vi "Execute FlatSeqOutTun Handle.vi"(6 "Menu Item Tag Suffix":string, 8 "错误输入（无错误）":errorcluster, 11 "平铺式顺序外部隧道输入":refnum<vi>) -> (0 "错误输出":errorcluster)   [LabVIEW 2020]
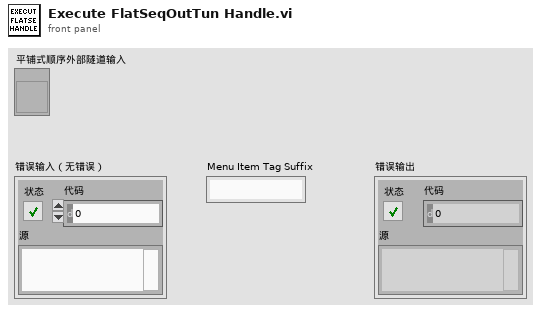
[diagram p1: front panel]
types:
  T1 = typedef "LVRectTypeDef.ctl" = cluster{"Left":i16, "Top":i16, "Right":i16, "Bottom":i16}
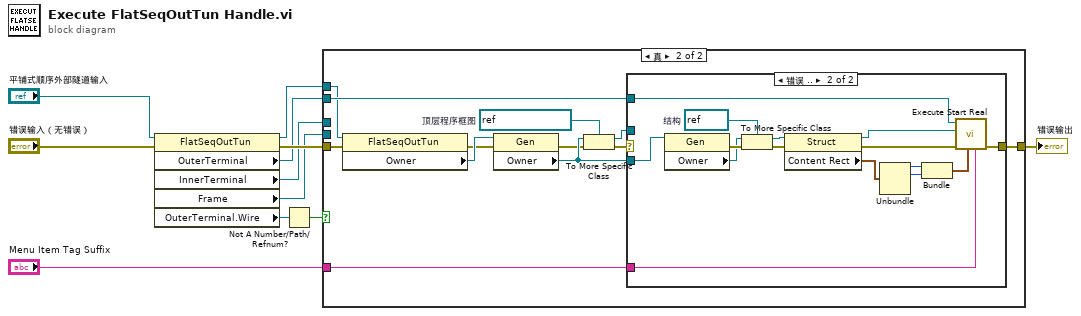
[diagram p0: block diagram]
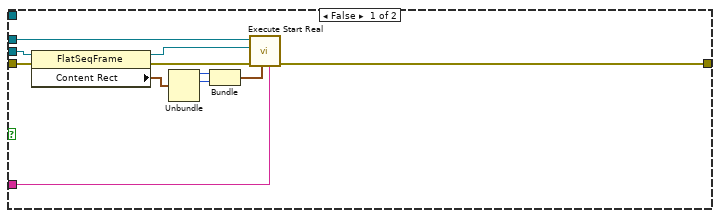
[diagram p2: hidden frame]
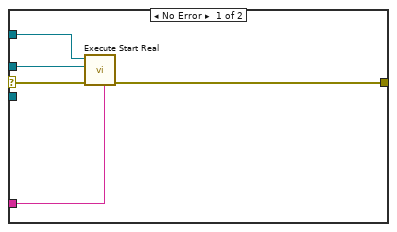
[diagram p3: hidden frame]
diagram:
  n1 = property class="FlatSeqOutTun"(reference="平铺式顺序外部隧道输入", error in="错误输入（无错误）") -> (reference out=w6:refnum<vi>, error out=w11:errorcluster, "OuterTerminal"=w2:refnum<vi>, "InnerTerminal"=w7:refnum<vi>, "Frame"=w8:refnum<vi>, "OuterTerminal.Wire"=w1:refnum<vi>)
  n2 = Not A Number/Path/Refnum?(number/path/refnum=w1) -> (NaN/Path/Refnum?=w4:bool)
  n3 = case shown="真" w4 {
    tunnel: w2 -> [_ w34]
    tunnel: "Menu Item Tag Suffix" -> [w16 w32]
    tunnel: w6 -> [_ w33]
    tunnel: w11 -> [w14 w31]
    tunnel: w7 -> [w15 _]
    tunnel: w8 -> [w22 _]
    tunnel: [w12 w25] -> w9
    frame False {
      n4 = property class="FlatSeqFrame"(reference=w22, error in=w14) -> (reference out=w21:refnum<vi>, error out=w13:errorcluster, "Content Rect"=w18:T1)
      n5 = Unbundle(w18) -> ("Left"=w20:i16, "Top"=w19:i16)  [unwired: 2 out]
      n6 = Bundle("Left"=w20, "Top"=w19) -> (w17:cluster{"Left":i16, "Top":i16})  [unwired: 1 in]
      n7 = call "Execute Start Real.vi"("Menu Item Tag Suffix"=w16, "相对位置原点"=w17, "错误输入（无错误）"=w13, "所有者引用句柄"=w21, "接线端输入"=w15) -> ("错误输出"=w12:errorcluster)  [unwired: 6 in]
    }
    frame True {
      w30 = refnum<vi> refnum  # 顶层程序框图
      n8 = property class="FlatSeqOutTun"(reference=w33, error in=w31) -> (error out=w23:errorcluster, "Owner"=w27:refnum<vi>)  [unwired: 1 out]
      n9 = property class="Gen"(reference=w27, error in=w23) -> (error out=w24:errorcluster, "Owner"=w26:refnum<vi>)  [unwired: 1 out]
      n10 = To More Specific Class(target class=w30, reference=w26, error in=w24) -> (specific class reference=w28:refnum<vi>, error out=w29:errorcluster)
      n11 = case shown="错误 .." w29 {
        selector: w29 -> [w39 _]
        tunnel: w28 -> [w38 _]
        tunnel: w34 -> [w37 w47]
        tunnel: w32 -> [w35 w41]
        tunnel: w26 -> [_ w44]
        tunnel: [w36 w42] -> w25
        frame No Error {
          n12 = call "Execute Start Real.vi"("Menu Item Tag Suffix"=w35, "错误输入（无错误）"=w39, "所有者引用句柄"=w38, "接线端输入"=w37) -> ("错误输出"=w36:errorcluster)  [unwired: 7 in]
        }
        frame Error {
          w54 = refnum<vi> refnum  # 结构
          n13 = property class="Gen"(reference=w44) -> (error out=w45:errorcluster, "Owner"=w43:refnum<vi>)  [unwired: 1 in, 1 out]
          n14 = To More Specific Class(target class=w54, reference=w43, error in=w45) -> (specific class reference=w52:refnum<vi>, error out=w53:errorcluster)
          n15 = property class="Struct"(reference=w52, error in=w53) -> (reference out=w46:refnum<vi>, error out=w48:errorcluster, "Content Rect"=w51:T1)
          n16 = Unbundle(w51) -> ("Left"=w50:i16, "Top"=w49:i16)  [unwired: 2 out]
          n17 = Bundle("Left"=w50, "Top"=w49) -> (w40:cluster{"Left":i16, "Top":i16})  [unwired: 1 in]
          n18 = call "Execute Start Real.vi"("Menu Item Tag Suffix"=w41, "相对位置原点"=w40, "错误输入（无错误）"=w48, "所有者引用句柄"=w46, "接线端输入"=w47) -> ("错误输出"=w42:errorcluster)  [unwired: 6 in]
        }
      }
    }
  }
  "错误输出" <- w9
